vi "Is Invalid.vi"(3 "error in (no error)":errorcluster, 4 "SQLite3LV Connection in":refnum<class "sqlite3.lvclass">) -> (0 "error out":errorcluster, 1 "not a database":bool)   [LabVIEW 2014, in "SQLite3LV.lvlib" / "sqlite3.lvclass"]
uses:
  sqlite3.lvclass
  sqlite3.lvclass/sqlite3.ctl
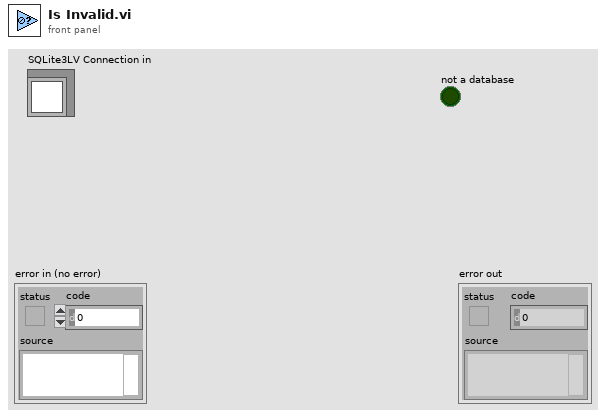
[diagram p1: front panel]
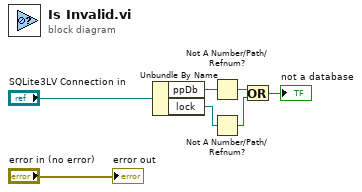
[diagram p0: block diagram]
diagram:
  n1 = Unbundle By Name("SQLite3LV Connection in") -> ("ppDb"=w2:refnum<data-value>, "lock"=w5:refnum<data-value>)
  n2 = Not A Number/Path/Refnum?(number/path/refnum=w2) -> (NaN/Path/Refnum?=w1:bool)
  n3 = Not A Number/Path/Refnum?(number/path/refnum=w5) -> (NaN/Path/Refnum?=w4:bool)
  n4 = Or(x=w1, y=w4) -> (x .or. y?=→"not a database":bool)
  "error out" <- "error in (no error)"
